vi "Set Mode.vi"(6 "Program No.":i32, 7 "Operation Mode":T1, 8 "error in (no error)":errorcluster, 10 "Address (0)":i32, 11 "VISA resource name":refnum<visa-resource-name>) -> (0 "error out":errorcluster, 3 "VISA resource name out":refnum<visa-resource-name>)   [LabVIEW 2016, in "Environment Chamber.lvlib" / "Climatic Chamber.lvlib"]
doc: "<b>Operation mode settings</B>\n\nMigrates to the specified operation mode.\n\n<b>Operation Modes:</b>\n- OFF\n- STANDBY\n- CONSTANT\n- RUN (Program No. must be specified)"
uses:
  Climatic Chamber.lvlib
  Private/Type Defs/Operation_Stop Mode Enum.ctl
panel:
  out "NACK":bool
  out "Error":bool
  out "ACK":bool
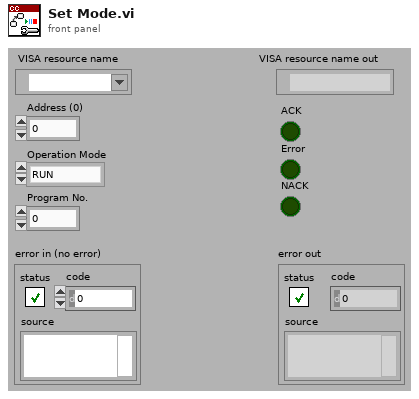
[diagram p1: front panel]
types:
  T1 = typedef "Environment Chamber.lvlib/Climatic Chamber.lvlib/Operation_Stop Mode Enum.ctl" = enum16{"RUN", "CONSTANT", "STANDBY", "OFF"}
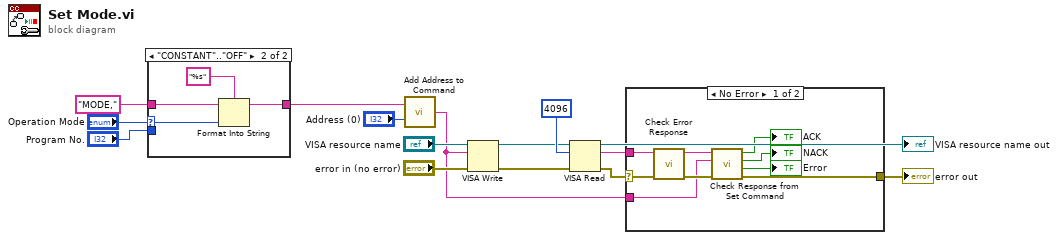
[diagram p0: block diagram]
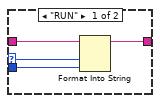
[diagram p2: hidden frame]
diagram:
  n1 = case shown="\"CONSTANT\"..\"OFF\"" "Operation Mode" {
    selector: "Operation Mode" -> [w17 w21]
    tunnel: "MODE," -> [w18 w23]
    tunnel: [w19 w22] -> w3
    tunnel: "Program No." -> [w16 _]
    frame "RUN" {
      n2 = Format Into String(initial string=w18, w17, w16) -> (resulting string=w19:string)  [unwired: 2 in, 1 out]
    }
    frame "CONSTANT".."OFF" {
      n3 = Format Into String(format string="%s", initial string=w23, w21) -> (resulting string=w22:string)  [unwired: 1 in, 1 out]
    }
  }
  n4 = call "Add Address to Command.vi"("Address (0)"="Address (0)", "Command"=w3) -> ("Command OUT"=w5:string)
  n5 = VISA Write(VISA resource name="VISA resource name", write buffer=w5, error in (no error)="error in (no error)") -> (VISA resource name out=w12:refnum<visa-resource-name>, error out=w11:errorcluster)  [unwired: 1 out]
  n6 = VISA Read(VISA resource name=w12, byte count=u32 4096, error in (no error)=w11) -> (VISA resource name out=→"VISA resource name out":refnum<visa-resource-name>, read buffer=w7:string, error out=w8:errorcluster)  [unwired: 1 out]
  n7 = case shown="No Error" w8 {
    selector: w8 -> [w31 w33]
    tunnel: w7 -> [w32 _]
    tunnel: [w27 w33] -> w6
    tunnel: w5 -> [w28 _]
    frame No Error {
      n8 = call "Check Error Response.vi"("error in (no error)"=w31, "read String"=w32) -> ("error out"=w30:errorcluster, "String out"=w29:string)  [unwired: 7 in, 1 out]
      n9 = call "Check Response from Set Command.vi"("error in (no error)"=w30, "Command"=w28, "Response"=w29) -> ("error out"=w27:errorcluster, "Error"=→"Error":bool, "NACK"=→"NACK":bool, "ACK"=→"ACK":bool)  [unwired: 5 in]
    }
    frame Error {
    }
  }
  "error out" <- w6
